vi "Set Temperature Covesion.vi"(8 "error in (no error)":errorcluster, 9 "Setpoint":dbl=30.0, 10 "Enable":bool=TRUE, 11 "VISA resource name":refnum<visa-resource-name>="COM6") -> (0 "error out":errorcluster)   [LabVIEW 2009]
panel:
  # "V1.02"
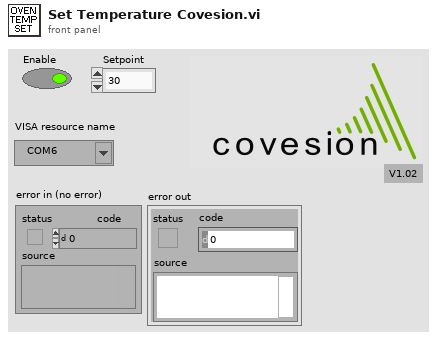
[diagram p1: front panel]
types:
  T1 = cluster{"Setpoint":u16, "pot range":dbl, "value":dbl, "pot offset":dbl, "X coeff deg/V":dbl, "Rate deg/V":dbl, "C coeff deg":dbl}
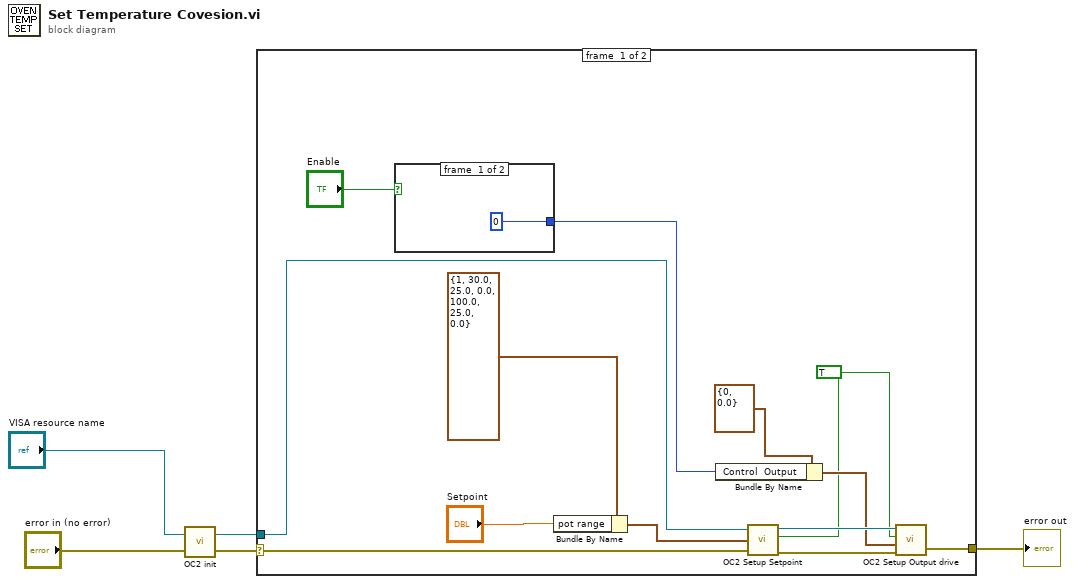
[diagram p0: block diagram]
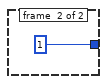
[diagram p2: hidden frame]
diagram:
  n1 = call "OC2 init.vi"("error in (no error)"="error in (no error)", "VISA resource name"="VISA resource name") -> ("error out"=w3:errorcluster, "duplicate VISA resource name"=w2:refnum<visa-resource-name>)
  n2 = case shown="No Error" w3 {
    selector: w3 -> [w15 w21]
    tunnel: w2 -> [w18 _]
    tunnel: [w9 w21] -> w1
    frame #0 {
      w6 = TRUE ("enable")
      n3 = case shown="False" "Enable" {
        tunnel: [u16 0 ("Control  Output") u16 1 ("Control  Output")] -> w7
        frame #0 {
        }
        frame #1 {
        }
      }
      n4 = Bundle By Name(cluster=T1 {"Setpoint"=1, "pot range"=30.0, "value"=25.0, "pot offset"=0.0, "X coeff deg/V"=100.0, "Rate deg/V"=25.0, "C coeff deg"=0.0} ("Setup setpoint values in"), "pot range"="Setpoint") -> (w16:T1)
      n5 = Bundle By Name(cluster=cluster{"Control  Output":u16, "Output %":dbl} {"Control  Output"=0, "Output %"=0.0} ("control output values"), "Control  Output"=w7) -> (w11:cluster{"Control  Output":u16, "Output %":dbl})
      n6 = call "OC2 Setup Setpoint.vi"("VISA resource name"=w18, "Setup setpoint values in"=w16, "error in (no error)"=w15, "enable"=w6) -> ("dup VISA resource name"=w13:refnum<visa-resource-name>, "error out"=w10:errorcluster)  [unwired: 1 out]
      n7 = call "OC2 Setup Output drive.vi"("error in (no error)"=w10, "control output values"=w11, "write control output"=w6, "VISA resource name"=w13) -> ("error out"=w9:errorcluster)  [unwired: 1 out]
    }
    frame #1 {
    }
  }
  "error out" <- w1
